vi "Postflight Position.vi"(4 "error in (no error)":errorcluster) -> (0 "error out":errorcluster, 3 "function return":i32)   [LabVIEW 2020, in "MPH16.lvlib"]
doc: "long PostflightPosition();"
uses:
  MPH16.lvlib
  ThorPinholeStepper.dll
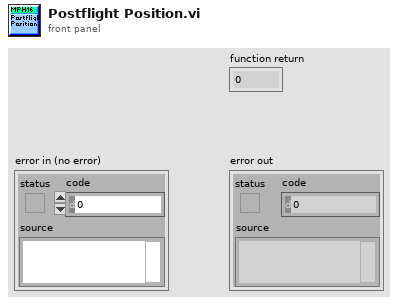
[diagram p1: front panel]
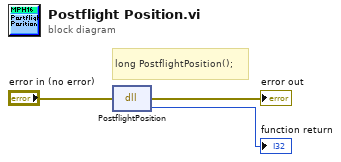
[diagram p0: block diagram]
diagram:
  # "long PostflightPosition();"
  n1 = dll-call lib="D:/software/TweezerTron Project/Instruments/Thorlabs/MPH_SDK/ThorPinholeStepper.*" fn="PostflightPosition"(error in="error in (no error)") -> (error out=→"error out":errorcluster, →"function return":i32)  [unwired: 2 in, 1 out]
